vi "CaseStructure Get Frames Output Assignements.vi"(11 "object ref":refnum<vi>) -> ()   [LabVIEW 2014]
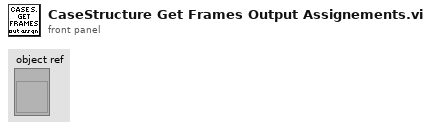
[diagram p1: front panel]
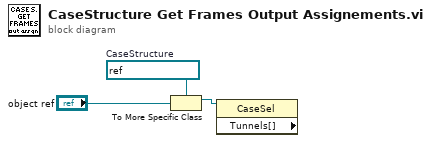
[diagram p0: block diagram]
diagram:
  w3 = refnum<vi> refnum  # CaseStructure
  n1 = To More Specific Class(target class=w3, reference="object ref") -> (specific class reference=w2:refnum<vi>)  [unwired: 1 in, 1 out]
  n2 = property class="CaseSel" props=["Tunnels[]"](reference=w2) -> ()  [unwired: 1 in, 3 out]
